vi "working_interface.vi"() -> ()   [LabVIEW 2011]
panel:
  in  "time unit":enum16{"s", "ms", "us", "ns"}(ring)=enum."us"
  in  "resolution":i32=100
  out "data in delay generator (s)":dbl[](array[numeric]) caption="delay array" min=0.0 max=2000.0 format="%.3f"
  in  "duration array":dbl[](array[numeric]) format="%.3f"
  in  "start time array":dbl[](array[numeric]) format="%.3f"
  out "Digital Waveform Graph":digitalwaveform(graph)
  in  "trigger":bool
  in  "write data":bool
  in  "read delay data":bool
  in  "VISA resource name":refnum<visa-resource-name>="TRIG"
  in  "stop":bool
  # "timing values are only relative,\n the absolute values are given in the\ndelay array!!!\n\nt0 and t can not be written to the device, t0 is always 0\nand  t is always the longest time + 25ns. However, t is \nused to display how long the nozzle is open to give a real \nrepresentation in the diagram (and only there). \nYou can change that time to pretty much any value, \nbut the nozzle itself is not controlled through the labview\n software. You have to set the time manually at the \nnozzle driver and ideally you should then enter that time\nfor t as well!\n\ndelay array index:\n0 - t0 = nozzle start (TTL) = 0\n1 - nozzle duration\n2 - power AMP START\n3 - power AMP STOP\n4 - AWG START (TTL)\n5 - AWG STOP (NA)\n6 - SWITCH ON \n7 - SWITCH OFF\n8 - OSC START (TTL)\n9 - OSC STOP (NA)\n\nTTL -> tool starts on rising flank\nof signal, hence the falling flank \nand the duration are not important!"
  # "delay array index:\n0 - to = nozzle start (TTL) = 0\n1 - t = nozzle duration\n2 - A = power AMP START\n3 - B = power AMP STOP\n4 - C = AWG START (TTL)\n5 - D = AWG STOP (NA)\n6 - E = SWITCH ON \n7 - F = SWITCH OFF\n8 - G = OSC START (TTL)\n9 - H = OSC STOP (NA)\n\nTTL -> tool starts on rising flank\nof signal, hence the falling flank \nand the duration are not important!"
  # "t0 is always 0"
  # "AWG must start after power AMP is on \nand while it is still on!"
  # "SWITCH must NOT switch ON before \npower AMP is off!"
  # "t0"
  # "t"
  # "A"
  # "B"
  # "C"
  # "D"
  # "E"
  # "F"
  # "G"
  # "H"
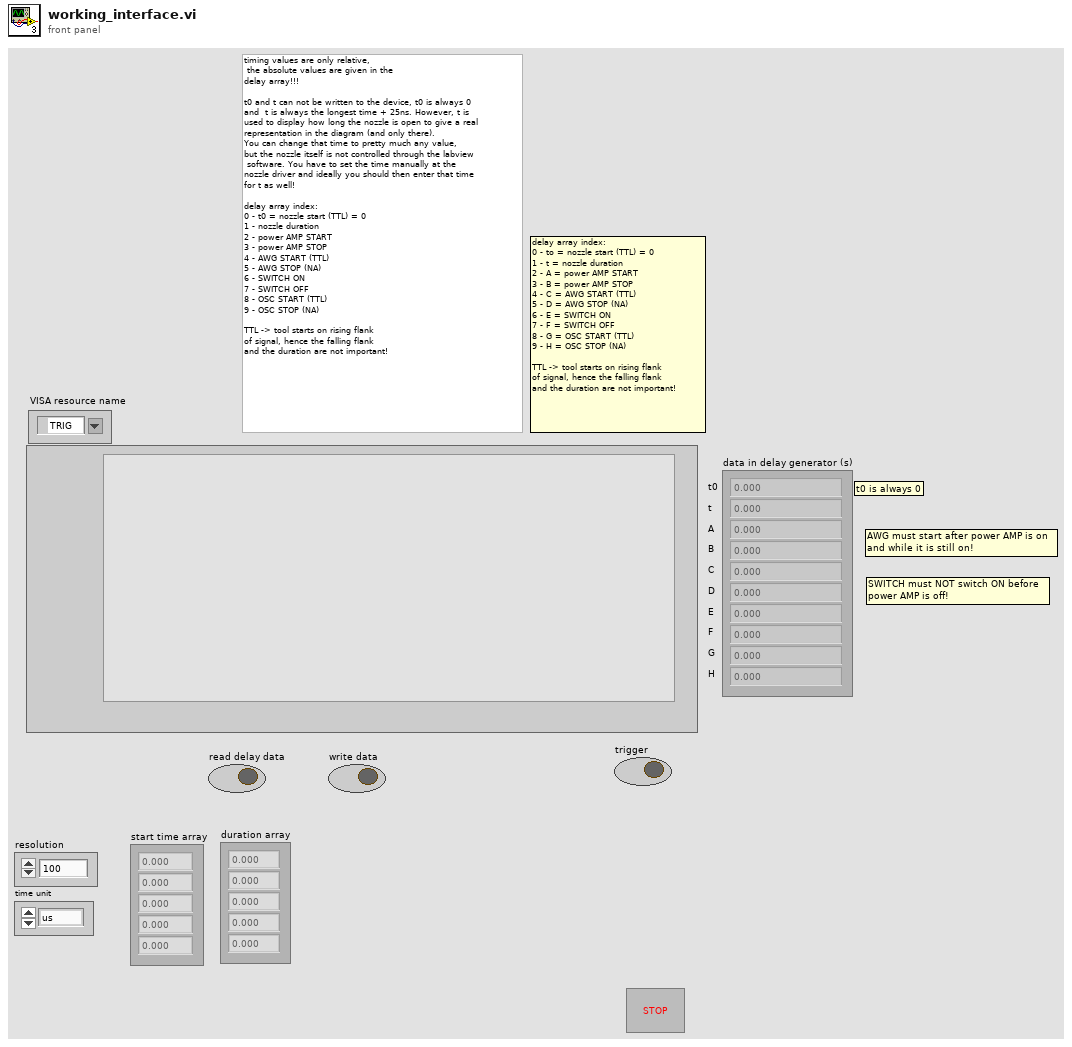
[diagram p1: front panel]
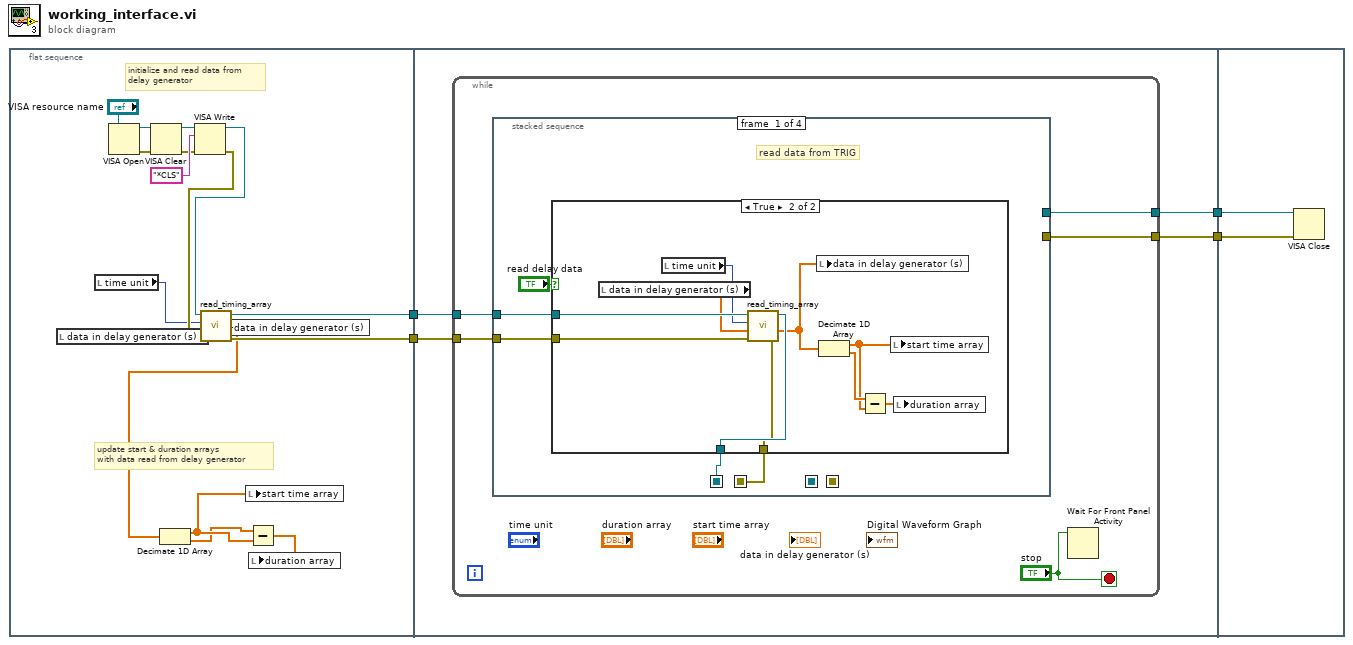
[diagram p0: block diagram]
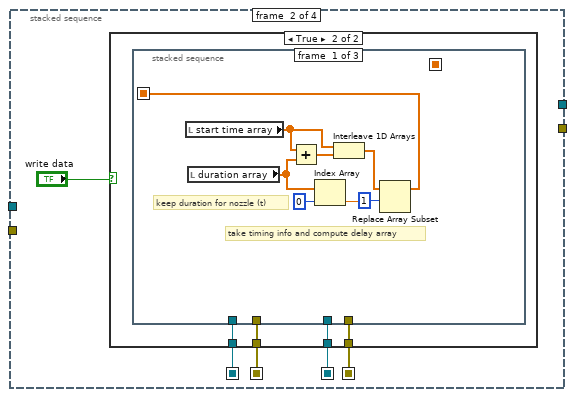
[diagram p3: hidden frame]
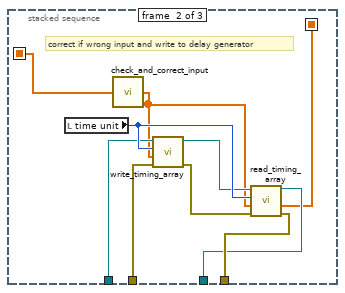
[diagram p5: hidden frame]
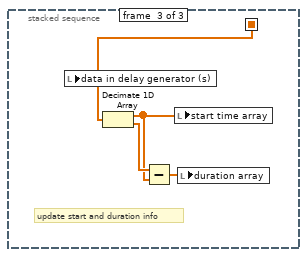
[diagram p6: hidden frame]
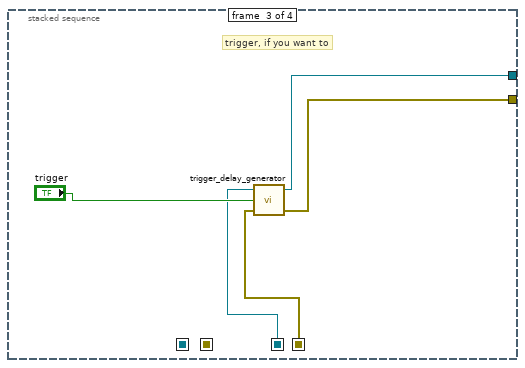
[diagram p7: hidden frame]
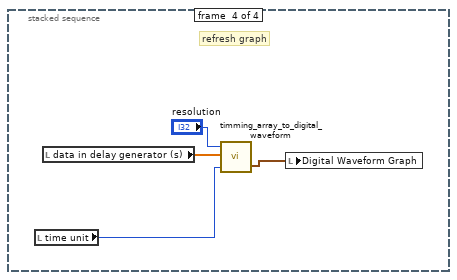
[diagram p8: hidden frame]
diagram:
  n1 = flat-sequence {
    tunnel: [w12] -> w4
    tunnel: [w13] -> w3
    tunnel: w4 -> [w24]
    tunnel: w3 -> [w23]
    tunnel: [w22] -> w2
    tunnel: [w21] -> w1
    tunnel: w2 -> [w90]
    tunnel: w1 -> [w89]
    frame #0 {
      # "update start & duration arrays \nwith data read from delay generator"
      # "initialize and read data from \ndelay generator"
      n2 = local read "data in delay generator (s)"() -> (w14:dbl[])
      n3 = local read "time unit"() -> (w6:enum16{"s", "ms", "us", "ns"})
      n4 = VISA Open(VISA resource name="VISA resource name") -> (VISA resource name=w17:refnum<visa-resource-name>, error out=w18:errorcluster)  [unwired: 4 in]
      n5 = VISA Clear(VISA resource name=w17, error in (no error)=w18) -> (VISA resource name out=w16:refnum<visa-resource-name>, error out=w15:errorcluster)
      n6 = VISA Write(VISA resource name=w16, write buffer="*CLS" ("Query 2"), error in (no error)=w15) -> (VISA resource name out=w10:refnum<visa-resource-name>, error out=w11:errorcluster)  [unwired: 1 out]
      n7 = call "read_timing_array.vi"("error in"=w11, "input array"=w14, "time unit"=w6, "VISA resource in"=w10) -> ("error out 2"=w13:errorcluster, "delay array"=w5:dbl[], "VISA resource out"=w12:refnum<visa-resource-name>)  [unwired: 1 in]
      n8 = Decimate 1D Array(w5) -> (w8:dbl[], w7:dbl[])
      n9 = local write "data in delay generator (s)"(w5) -> ()
      n10 = local write "start time array"(w8) -> ()
      n11 = Subtract(x=w7, y=w8) -> (x-y=w9:dbl[])
      n12 = local write "duration array"(w9) -> ()
    }
    frame #1 {
      n13 = while {
        tunnel: w23 -> [w27]
        tunnel: [w29] -> w22
        tunnel: [w28] -> w21
        tunnel: w24 -> [w25]
        stop <- "stop" stop-if-true
        n14 = stacked-sequence {
          seq-local: [w32 _ _ _] -> [_ w48 _ _]
          seq-local: [w31 _ _ _] -> [_ w47 _ _]
          seq-local: [_ w50 _ _] -> [_ _ w81 _]
          seq-local: [_ w49 _ _] -> [_ _ w82 _]
          tunnel: w25 -> [w34 _ _ _]
          tunnel: w27 -> [w33 _ _ _]
          tunnel: [_ _ w80 _] -> w28
          tunnel: [_ _ w84 _] -> w29
          frame #0 {
            # "read data from TRIG"
            n15 = case shown="True" "read delay data" {
              tunnel: w34 -> [w35 w46]
              tunnel: w33 -> [w36 w45]
              tunnel: [w35 w44] -> w32
              tunnel: [w36 w43] -> w31
              frame False {
              }
              frame True {
                n16 = local read "data in delay generator (s)"() -> (w42:dbl[])
                n17 = local read "time unit"() -> (w41:enum16{"s", "ms", "us", "ns"})
                n18 = call "read_timing_array.vi"("error in"=w45, "input array"=w42, "time unit"=w41, "VISA resource in"=w46) -> ("error out 2"=w43:errorcluster, "delay array"=w38:dbl[], "VISA resource out"=w44:refnum<visa-resource-name>)  [unwired: 1 in]
                n19 = local write "data in delay generator (s)"(w38) -> ()
                n20 = Decimate 1D Array(w38) -> (w37:dbl[], w39:dbl[])
                n21 = Subtract(x=w39, y=w37) -> (x-y=w40:dbl[])
                n22 = local write "start time array"(w37) -> ()
                n23 = local write "duration array"(w40) -> ()
              }
            }
          }
          frame #1 {
            n24 = case shown="True" "write data" {
              tunnel: [w53 w54] -> w50
              tunnel: [w52 w57] -> w49
              tunnel: w48 -> [w53 w56]
              tunnel: w47 -> [w52 w55]
              frame False {
              }
              frame True {
                n25 = stacked-sequence {
                  seq-local: [w58 _ _] -> [_ w67 _]
                  seq-local: [_ w66 _] -> [_ _ w77]
                  tunnel: [_ w75 _] -> w57
                  tunnel: w56 -> [_ w73 _]
                  tunnel: w55 -> [_ w72 _]
                  tunnel: [_ w69 _] -> w54
                  frame #0 {
                    # "take timing info and compute delay array"
                    # "keep duration for nozzle (t)"
                    n26 = local read "start time array"() -> (w64:dbl[])
                    n27 = local read "duration array"() -> (w63:dbl[])
                    n28 = Add(x=w64, y=w63) -> (x+y=w65:dbl[])
                    n29 = Index Array(array=w63, index=0) -> (element=w59:dbl)
                    n30 = Interleave 1D Arrays(w64, w65) -> (w61:dbl[])
                    n31 = Replace Array Subset(array=w61, new element=w59, index=1) -> (w58:dbl[])
                  }
                  frame #1 {
                    # "correct if wrong input and write to delay generator"
                    n32 = local read "time unit"() -> (w74:enum16{"s", "ms", "us", "ns"})
                    n33 = call "check_and_correct_input.vi"("delay array"=w67) -> ("corrrected delay array"=w68:dbl[])  [unwired: 4 in]
                    n34 = call "write_timing_array.vi"("error in"=w72, "delay array"=w68, "time unit"=w74, "VISA resource in"=w73) -> ("error out 2"=w70:errorcluster, "VISA resource out"=w71:refnum<visa-resource-name>)  [unwired: 2 in]
                    n35 = call "read_timing_array.vi"("error in"=w70, "input array"=w68, "time unit"=w74, "VISA resource in"=w71) -> ("error out 2"=w75:errorcluster, "delay array"=w66:dbl[], "VISA resource out"=w69:refnum<visa-resource-name>)  [unwired: 1 in]
                  }
                  frame #2 {
                    # "update start and duration info"
                    n36 = local write "data in delay generator (s)"(w77) -> ()
                    n37 = Decimate 1D Array(w77) -> (w76:dbl[], w79:dbl[])
                    n38 = Subtract(x=w79, y=w76) -> (x-y=w78:dbl[])
                    n39 = local write "start time array"(w76) -> ()
                    n40 = local write "duration array"(w78) -> ()
                  }
                }
              }
            }
          }
          frame #2 {
            # "trigger, if you want to"
            n41 = call "trigger_delay_generator.vi"("error in (no error)"=w82, "Boolean"="trigger", "VISA resource name"=w81) -> ("error out"=w80:errorcluster, "VISA resource name 2"=w84:refnum<visa-resource-name>)  [unwired: 1 in]
          }
          frame #3 {
            # "refresh graph"
            n42 = local read "time unit"() -> (w85:enum16{"s", "ms", "us", "ns"})
            n43 = local read "data in delay generator (s)"() -> (w88:dbl[])
            n44 = call "timming_array_to_digital_waveform.vi"("time unit"=w85, "delay array"=w88, "resolution"="resolution") -> ("digital waveform"=w87:digitalwaveform)  [unwired: 1 in]
            n45 = local write "Digital Waveform Graph"(w87) -> ()
          }
        }
        n46 = Wait For Front Panel Activity(3:"stop") -> ()  [unwired: 2 in, 1 out]
      }
    }
    frame #2 {
      n47 = VISA Close(VISA resource name=w90, error in (no error)=w89) -> ()  [unwired: 1 out]
    }
  }
